vi "Get Next Command ID.vi"(8 "error in (no error)":errorcluster, 11 "Command Processor Actor in":refnum<class "Command Processor Actor.lvclass">) -> (0 "error out":errorcluster, 2 "Next Command ID":u32, 3 "Command Processor Actor out":refnum<class "Command Processor Actor.lvclass">)   [LabVIEW 2014, in "Robot Actor Framework.lvlib" / "Command Processor Actor.lvlib" / "Command Processor Actor.lvclass"]
uses:
  Command Processor Actor.lvclass
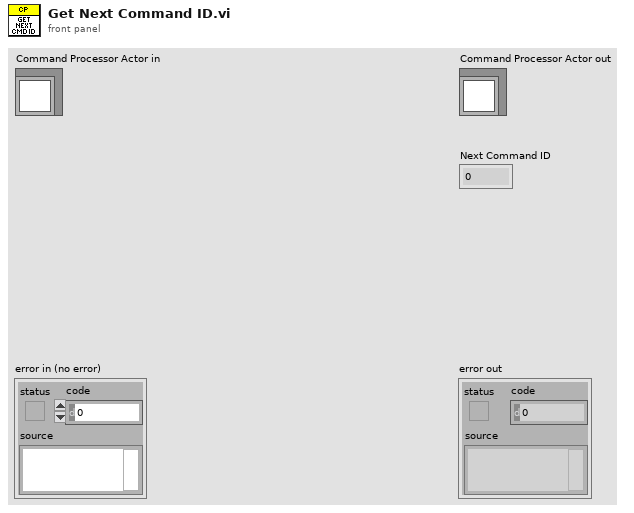
[diagram p1: front panel]
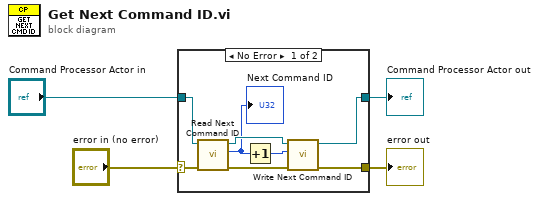
[diagram p0: block diagram]
diagram:
  n1 = case shown="No Error" "error in (no error)" {
    selector: "error in (no error)" -> [w7 w14]
    tunnel: [w5 w14] -> w3
    tunnel: [w10 w13] -> w1
    tunnel: "Command Processor Actor in" -> [w11 w13]
    frame No Error {
      n2 = call-dynamic "Read Next Command ID.vi"("error in (no error)"=w7, "Command Processor Actor in"=w11) -> ("error out"=w6:errorcluster, "Next Command ID"=w9:u32, "Command Processor Actor out"=w12:refnum<class "Command Processor Actor.lvclass">)  [unwired: 7 in]
      "Next Command ID" <- w9
      n3 = Increment(x=w9) -> (x+1=w8:u32)
      n4 = call-dynamic "Write Next Command ID.vi"("error in (no error)"=w6, "Next Command ID"=w8, "Command Processor Actor in"=w12) -> ("error out"=w5:errorcluster, "Command Processor Actor out"=w10:refnum<class "Command Processor Actor.lvclass">)  [unwired: 7 in]
    }
    frame Error {
    }
  }
  "error out" <- w3
  "Command Processor Actor out" <- w1
